vi "Generator DC Sweep Manager.vi"(8 "error in (no error)":errorcluster, 10 "sweep index":i32=-1, 11 "Instrument.DAQ in":refnum<class "Instrument.DAQ.lvclass">) -> (0 "error out":errorcluster, 2 "Waveform []":waveform(dbl)[](array[waveform]), 3 "Instrument.DAQ out":refnum<class "Instrument.DAQ.lvclass">)   [LabVIEW 2019, in "Instrument.DAQ.lvclass"]
uses:
  Instrument.DAQ.lvclass
  Instrument.DAQ.lvclass/Instrument.DAQ.ctl
panel:
  out "time":dbl
  out "sweeping":dbl
  out "start sweep time":timestamp
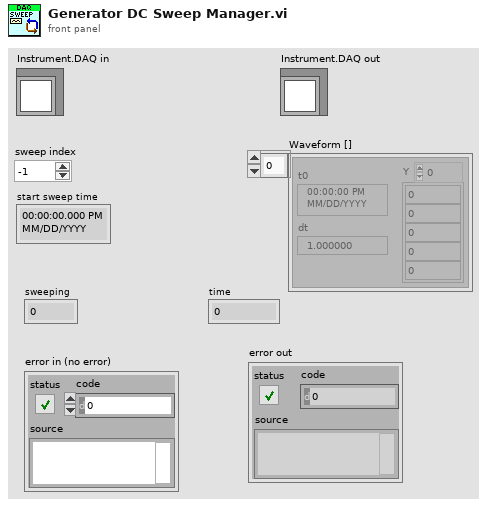
[diagram p1: front panel]
types:
  T1 = typedef "Instrument.DAQ.lvclass/AO.Channel--Cluster--Array.ctl" = T2[]
  T2 = typedef "Instrument.DAQ.lvclass/AO.Channel--Cluster.ctl" = cluster{"Enable?":bool, "Channel":i32, "Amplitude":dbl, "Offset":dbl, "Frequency":dbl, "Phase":dbl, "Function":T3, "Sweeping?":bool}
  T3 = typedef "Instrument.DAQ.lvclass/AO.Channel.Function--Enum.ctl" = enum16{"Sine", "Triangle", "Square"}
  T4 = typedef "Instrument.DAQ.lvclass/Sweep.Channel--Cluster--Array.ctl" = T5[]
  T5 = typedef "Instrument.DAQ.lvclass/Sweep.Channel--Cluster.ctl" = cluster{"Enable?":bool, "Channel":u16, "Start":dbl, "End":dbl, "Pattern":T6, "Table":dbl[]}
  T6 = typedef "Instrument.DAQ.lvclass/Sweep.Pattern--Enum.ctl" = enum16{"Ramp /", "Ramp /\\", "Smooth Ramp _/", "Smooth Ramp _/\\_", "Table"}
  T7 = typedef "Instrument.DAQ.lvclass/DAQ.Sampling.Sampling--Cluster.ctl" = cluster{"Fs":dbl, "#s":i32}
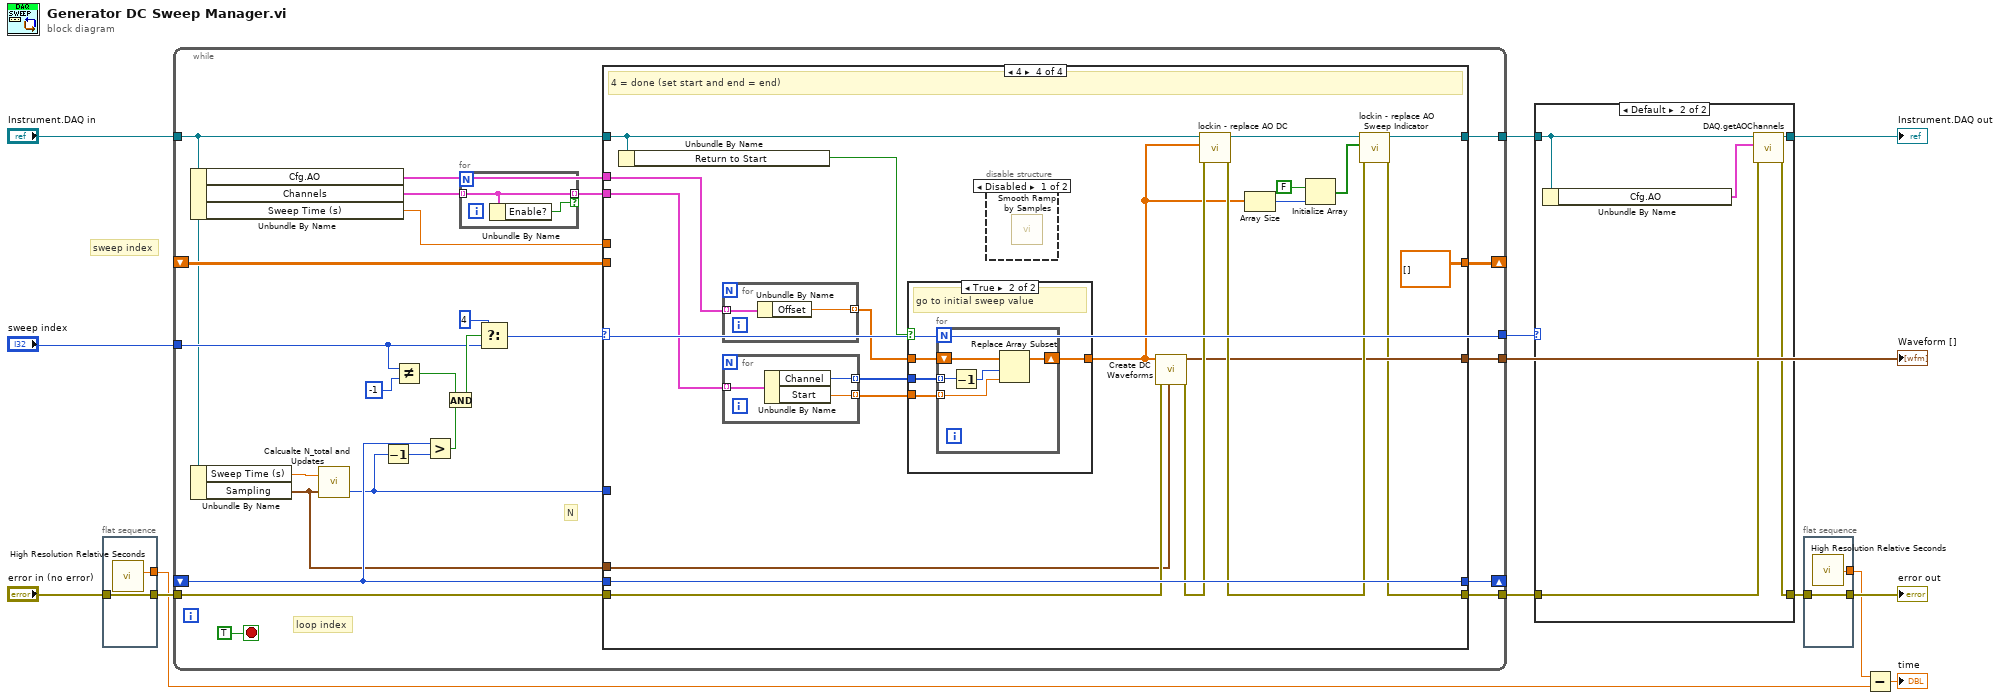
[diagram p0: block diagram]
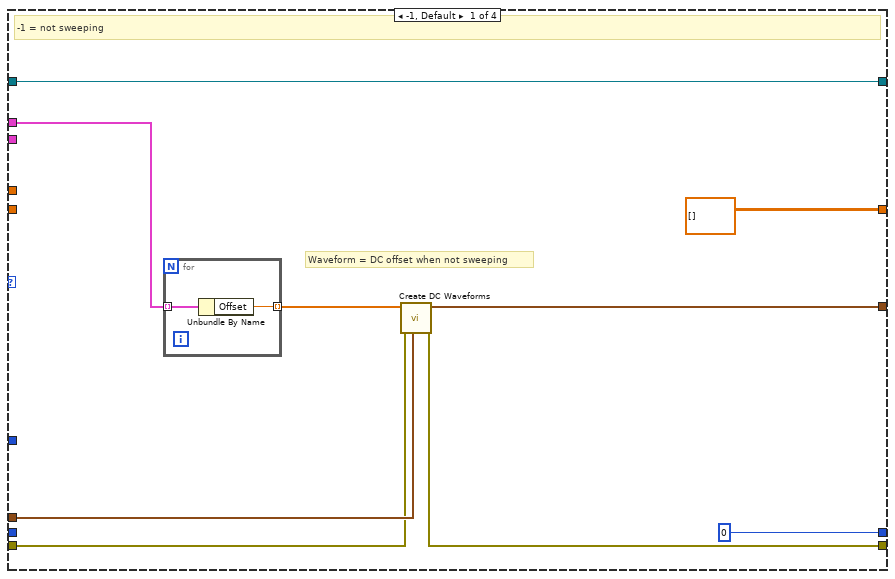
[diagram p3: hidden frame]
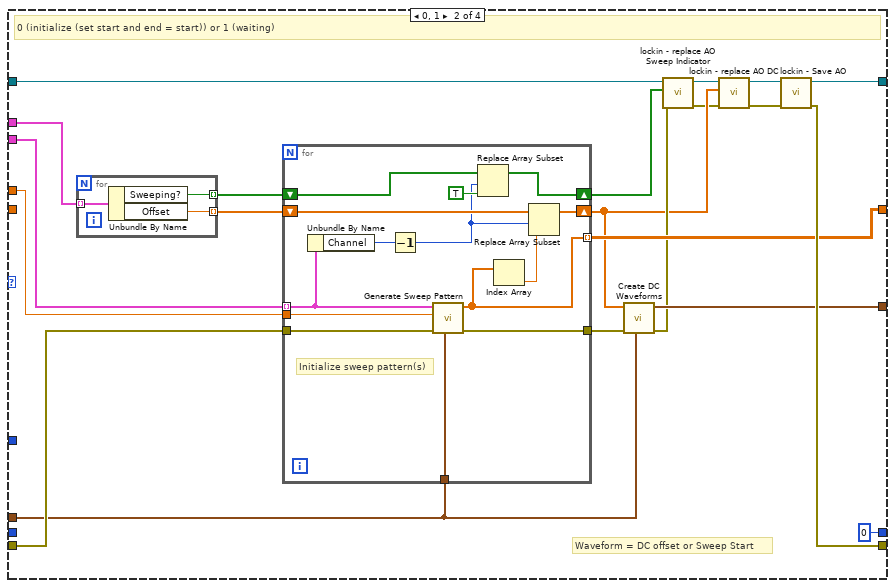
[diagram p4: hidden frame]
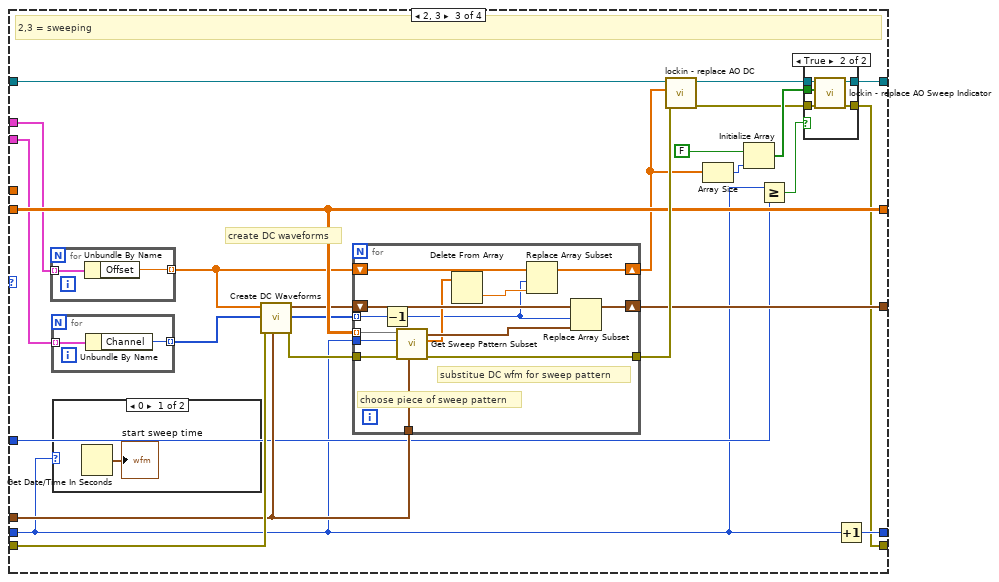
[diagram p5: hidden frame]
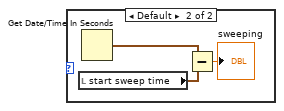
[diagram p6: hidden frame]
diagram:
  # "sweep index"
  n1 = flat-sequence {
    tunnel: "error in (no error)" -> [w16]
    tunnel: [w16] -> w11
    tunnel: [w15] -> w9
    frame #0 {
      n2 = call <vilib>:"High Resolution Relative Seconds.vi"() -> ("relative seconds"=w15:dbl)
    }
  }
  n3 = while {
    tunnel: "sweep index" -> [w25]
    shift-right: [w41] -> _
    shift-left: _ -> [w36]
    tunnel: [w39] -> w2
    tunnel: "Instrument.DAQ in" -> [w22]
    tunnel: w11 -> [w38]
    tunnel: [w37] -> w4
    shift-right: [w33] -> _
    shift-left: _ -> [w31]
    tunnel: [w34] -> w7
    tunnel: [w18] -> w1
    stop <- TRUE stop-if-true
    # "N"
    # "loop index"
    n4 = Unbundle By Name(w22) -> ("Cfg.AO"=w21:T1, "Channels"=w20:T4, "Sweep Time (s)"=w17:dbl)
    n5 = Unbundle By Name(w22) -> ("Sweep Time (s)"=w30:dbl, "Sampling"=w29:T7)
    n6 = call "Calcualte N_total and Updates.vi"("Configuration.DAQ.Sampling.Sampling"=w29, "Sweep Time (s)"=w30) -> ("Updates"=w24:i32)  [unwired: 1 out]
    n7 = Decrement(x=w24) -> (x-1=w23:i32)
    n8 = Not Equal?(x=w25, y=-1 ("x")) -> (x != y?=w27:bool)
    n9 = Greater?(x=w36, y=w23) -> (0:w35:bool)
    n10 = And(x=w27, y=w35) -> (x .and. y?=w28:bool)
    n11 = for {
      tunnel: w20 -> [w43] mode=indexing
      tunnel: [w43] -> w19 mode=indexing if=w42
      n12 = Unbundle By Name(w43) -> ("Enable?"=w42:bool)
    }
    n13 = Select(t=4, s=w28, f=w25) -> (s? t:f=w18:i32)
    n14 = case shown="4" w18 {
      tunnel: [0 0 w116 w165] -> w41
      tunnel: w36 -> [_ _ w94 w165]
      tunnel: w24 -> [_ _ w98 _]
      tunnel: [w46 w74 w103 w164] -> w39
      tunnel: w38 -> [w49 w70 w112 w161]
      tunnel: [w48 w73 w93 w150] -> w37
      tunnel: w29 -> [w50 w67 w110 w159]
      tunnel: [w47 w68 w108 w158] -> w34
      tunnel: [dbl[][] [] ("Sweep Pattern") w71 w114 dbl[][] [] ("Sweep Pattern")] -> w33
      tunnel: w31 -> [_ _ w114 _]
      tunnel: w22 -> [w46 w58 w107 w146]
      tunnel: w21 -> [w44 w56 w97 w147]
      tunnel: w19 -> [_ w55 w96 w153]
      tunnel: w17 -> [_ w57 _ _]
      frame -1, Default {
        # "Waveform = DC offset when not sweeping"
        # "-1 = not sweeping"
        n15 = for {
          tunnel: w44 -> [w54] mode=indexing
          tunnel: [w53] -> w45 mode=indexing
          n16 = Unbundle By Name(w54) -> ("Offset"=w53:dbl)
        }
        n17 = call "Create DC Waveforms.vi"("sampling"=w50, "error in (no error)"=w49, "DC (V)"=w45) -> ("Error out"=w48:errorcluster, "Waveforms []"=w47:waveform(dbl)[])  [unwired: 7 in]
      }
      frame 0, 1 {
        # "Waveform = DC offset or Sweep Start"
        # "0 (initialize (set start and end = start)) or 1 (waiting)"
        n18 = for {
          tunnel: [w78] -> w69 mode=indexing
          tunnel: [w77] -> w64 mode=indexing
          tunnel: w56 -> [w76] mode=indexing
          n19 = Unbundle By Name(w76) -> ("Sweeping?"=w77:bool, "Offset"=w78:dbl)
        }
        n20 = for {
          shift-right: [w91] -> w63
          shift-left: w69 -> [w92]
          shift-right: [w90] -> w72
          shift-left: w64 -> [w86]
          tunnel: w57 -> [w82]
          tunnel: w70 -> [w83]
          tunnel: w67 -> [w89]
          tunnel: [w85] -> w71 mode=indexing
          tunnel: [w87] -> w66
          tunnel: w55 -> [w81] mode=indexing
          # "Initialize sweep pattern(s)"
          n21 = Unbundle By Name(w81) -> ("Channel"=w79:u16)
          n22 = Decrement(x=w79) -> (x-1=w80:u16)
          n23 = call "Generate Sweep Pattern.vi"("Configuration.DAQ.Sampling.Sampling"=w89, "error in (no error)"=w83, "Sweep Lockin Time (s)"=w82, "sweep cluster"=w81) -> ("error out"=w87:errorcluster, "Sweep Pattern out"=w85:dbl[])  [unwired: 6 in]
          n24 = Replace Array Subset(array=w86, new element=TRUE ("new element/subarray"), index=w80) -> (w90:bool[])
          n25 = Index Array(array=w85) -> (element=w84:dbl)  [unwired: 1 in]
          n26 = Replace Array Subset(array=w92, new element=w84, index=w80) -> (w91:dbl[])
        }
        n27 = call "Create DC Waveforms.vi"("sampling"=w67, "error in (no error)"=w66, "DC (V)"=w63) -> ("Error out"=w65:errorcluster, "Waveforms []"=w68:waveform(dbl)[])  [unwired: 7 in]
        n28 = call "lockin - replace AO Sweep Indicator.vi"("error in (no error)"=w65, "Channels: AO.Sweeping?"=w72, "Instrument.DAQ"=w58) -> ("error out"=w60:errorcluster, "Instrument.DAQout"=w61:refnum<class "Instrument.DAQ.lvclass">)  [unwired: 7 in]
        n29 = call "lockin - replace AO DC.vi"("error in (no error)"=w60, "AO.DC (V)"=w63, "Instrument.DAQ"=w61) -> ("error out"=w59:errorcluster, "Instrument.DAQ out"=w62:refnum<class "Instrument.DAQ.lvclass">)  [unwired: 7 in]
        n30 = call "lockin - Save AO.vi"("error in (no error)"=w59, "Instrument.DAQ"=w62) -> ("error out"=w73:errorcluster, "Instrument.DAQ out"=w74:refnum<class "Instrument.DAQ.lvclass">)  [unwired: 8 in]
      }
      frame 2, 3 {
        # "create DC waveforms"
        # "2,3 = sweeping"
        n31 = for {
          tunnel: [w120] -> w109 mode=indexing
          tunnel: w97 -> [w119] mode=indexing
          n32 = Unbundle By Name(w119) -> ("Offset"=w120:dbl)
        }
        n33 = for {
          tunnel: [w118] -> w95 mode=indexing
          tunnel: w96 -> [w117] mode=indexing
          n34 = Unbundle By Name(w117) -> ("Channel"=w118:u16)
        }
        n35 = case shown="0" w94 {
          frame 0 {
            n36 = Get Date/Time In Seconds() -> (seconds since 1Jan1904=→"start sweep time":timestamp)
          }
          frame Default {
            n37 = local read "start sweep time"() -> (w123:timestamp)
            n38 = Get Date/Time In Seconds() -> (seconds since 1Jan1904=w122:timestamp)
            n39 = Subtract(x=w122, y=w123) -> (x-y=→"sweeping":dbl)
          }
        }
        n40 = call "Create DC Waveforms.vi"("sampling"=w110, "error in (no error)"=w112, "DC (V)"=w109) -> ("Error out"=w111:errorcluster, "Waveforms []"=w113:waveform(dbl)[])  [unwired: 7 in]
        n41 = for {
          tunnel: w110 -> [w141]
          tunnel: w114 -> [w145] mode=indexing
          tunnel: w94 -> [w144]
          tunnel: w111 -> [w143]
          tunnel: [w142] -> w115
          shift-right: [w138] -> w108
          shift-left: w113 -> [w140]
          shift-right: [w136] -> w101
          shift-left: w109 -> [w137]
          tunnel: w95 -> [w133] mode=indexing
          # "substitue DC wfm for sweep pattern"
          # "choose piece of sweep pattern"
          n42 = Decrement(x=w133) -> (x-1=w132:u16)
          n43 = call "Get Sweep Pattern Subset.vi"("Configuration.DAQ.Sampling.Sampling"=w141, "error in (no error)"=w143, "index"=w144, "Sweep Pattern"=w145) -> ("error out"=w142:errorcluster, "Pattern Subset"=w135:dbl[], "output waveform"=w139:waveform(dbl))  [unwired: 5 in]
          n44 = Delete From Array(array=w135) -> (deleted portion=w134:dbl)  [unwired: 2 in, 1 out]
          n45 = Replace Array Subset(array=w137, new element=w134, index=w132) -> (w136:dbl[])
          n46 = Replace Array Subset(array=w140, new element=w139, index=w132) -> (w138:waveform(dbl)[])
        }
        n47 = call "lockin - replace AO DC.vi"("error in (no error)"=w115, "AO.DC (V)"=w101, "Instrument.DAQ"=w107) -> ("error out"=w100:errorcluster, "Instrument.DAQ out"=w104:refnum<class "Instrument.DAQ.lvclass">)  [unwired: 7 in]
        n48 = Array Size(array=w101) -> (size(s)=w102:i32)
        n49 = Initialize Array(FALSE, w102) -> (w105:bool[])
        n50 = Greater Or Equal?(x=w94, y=w98) -> (x >= y?=w99:bool)
        n51 = case shown="True" w99 {
          tunnel: w105 -> [_ w131]
          tunnel: w104 -> [w126 w130]
          tunnel: [w126 w129] -> w103
          tunnel: w100 -> [w125 w128]
          tunnel: [w125 w127] -> w93
          frame False {
          }
          frame True {
            n52 = call "lockin - replace AO Sweep Indicator.vi"("error in (no error)"=w128, "Channels: AO.Sweeping?"=w131, "Instrument.DAQ"=w130) -> ("error out"=w127:errorcluster, "Instrument.DAQout"=w129:refnum<class "Instrument.DAQ.lvclass">)  [unwired: 7 in]
          }
        }
        n53 = Increment(x=w94) -> (x+1=w116:i32)
      }
      frame 4 {
        # "4 = done (set start and end = end)"
        n54 = Unbundle By Name(w146) -> ("Return to Start"=w148:bool)
        n55 = for {
          tunnel: [w168] -> w152 mode=indexing
          tunnel: w147 -> [w167] mode=indexing
          n56 = Unbundle By Name(w167) -> ("Offset"=w168:dbl)
        }
        n57 = for {
          tunnel: [w171] -> w166 mode=indexing
          tunnel: [w170] -> w151 mode=indexing
          tunnel: w153 -> [w169] mode=indexing
          n58 = Unbundle By Name(w169) -> ("Channel"=w170:u16, "Start"=w171:dbl)
        }
        n59 = case shown="True" w148 {
          tunnel: w166 -> [_ w176]
          tunnel: w151 -> [_ w175]
          tunnel: w152 -> [w172 w174]
          tunnel: [w172 w173] -> w149
          frame False {
            # "remain at current value of DC"
          }
          frame True {
            # "go to initial sweep value"
            n60 = for {
              shift-right: [w179] -> w173
              shift-left: w174 -> [w181]
              tunnel: w176 -> [w180] mode=indexing
              tunnel: w175 -> [w178] mode=indexing
              n61 = Decrement(x=w178) -> (x-1=w177:u16)
              n62 = Replace Array Subset(array=w181, new element=w180, index=w177) -> (w179:dbl[])
            }
          }
        }
        n63 = disable-structure shown="Disabled" {
          frame Disabled {
            n64 = call "Smooth Ramp by Samples.vi"() -> ()  [unwired: 10 in, 2 out]
          }
          frame Enabled {
          }
        }
        n65 = call "Create DC Waveforms.vi"("sampling"=w159, "error in (no error)"=w161, "DC (V)"=w149) -> ("Error out"=w160:errorcluster, "Waveforms []"=w158:waveform(dbl)[])  [unwired: 7 in]
        n66 = call "lockin - replace AO DC.vi"("error in (no error)"=w160, "AO.DC (V)"=w149, "Instrument.DAQ"=w146) -> ("error out"=w162:errorcluster, "Instrument.DAQ out"=w163:refnum<class "Instrument.DAQ.lvclass">)  [unwired: 7 in]
        n67 = Array Size(array=w149) -> (size(s)=w156:i32)
        n68 = Initialize Array(FALSE, w156) -> (w155:bool[])
        n69 = call "lockin - replace AO Sweep Indicator.vi"("error in (no error)"=w162, "Channels: AO.Sweeping?"=w155, "Instrument.DAQ"=w163) -> ("error out"=w150:errorcluster, "Instrument.DAQout"=w164:refnum<class "Instrument.DAQ.lvclass">)  [unwired: 7 in]
      }
    }
  }
  "Waveform []" <- w7
  n70 = case shown="Default" w1 {
    tunnel: [w183 w188] -> w5
    tunnel: w4 -> [w182 w187]
    tunnel: [w182 w186] -> w3
    tunnel: w2 -> [w183 w185]
    frame -1 {
    }
    frame Default {
      n71 = Unbundle By Name(w185) -> ("Cfg.AO"=w184:T1)
      n72 = call "DAQ.getAOChannels.vi"("error in (no error)"=w187, "Channels: AO"=w184, "Instrument.DAQ"=w185) -> ("error out"=w186:errorcluster, "Instrument.DAQ out"=w188:refnum<class "Instrument.DAQ.lvclass">)  [unwired: 7 in]
    }
  }
  "Instrument.DAQ out" <- w5
  n73 = flat-sequence {
    tunnel: w3 -> [w190]
    tunnel: [w190] -> w10
    tunnel: [w189] -> w6
    frame #0 {
      n74 = call <vilib>:"High Resolution Relative Seconds.vi"() -> ("relative seconds"=w189:dbl)
    }
  }
  n75 = Subtract(x=w6, y=w9) -> (x-y=→"time":dbl)
  "error out" <- w10
